vi "AboutLS1.vi"(6 "error in (no error)":errorcluster caption="entrée d'erreur (pas d'erreur)") -> (0 "error out":errorcluster caption="sortie d'erreur")   [LabVIEW 2012]
doc: "Ce Vi affiche des informations sur le programme d'Absorptions Transitoire"
panel:
  in  "OK Button":bool
  # "LabScan V1.0"
  # "Crée par : Gabriel Laliberté\nLaboratoire de Spectroscopie\nUniversité de Sherbrooke\nAoût 2017\n\nMontage:\nPompe Sonde"
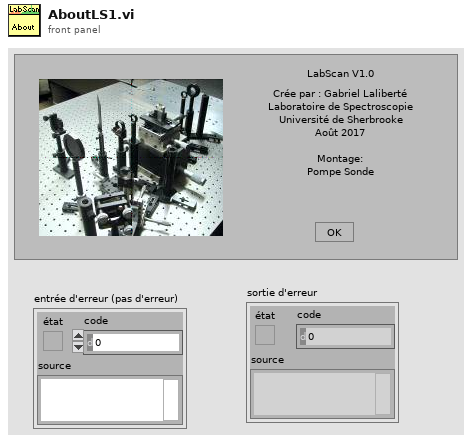
[diagram p1: front panel]
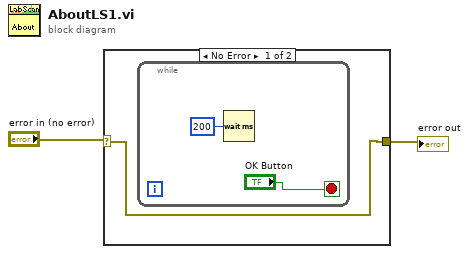
[diagram p0: block diagram]
diagram:
  n1 = case shown="No Error" "error in (no error)" {
    selector: "error in (no error)" -> [w3 w6]
    tunnel: [w3 w6] -> w1
    frame No Error {
      n2 = while {
        stop <- "OK Button" stop-if-true
        n3 = Wait (ms)(milliseconds to wait=u32 200) -> ()  [unwired: 1 out]
      }
    }
    frame Error {
    }
  }
  "error out" <- w1
